vi "write_signal.vi"(6 "Experiment Settings ID":i32, 7 "Index":i32, 8 "error in":errorcluster, 9 "File Name":string="\\", 10 "Save Path":path, 11 "Signal array":T1[](array[typedef])) -> (0 "error out":errorcluster)   [LabVIEW 2012]
uses:
  Public API/Signal.ctl
  Role ID.ctl
  Hardware ID.ctl
panel:
  out "concatenated string":string
  # "Signal"
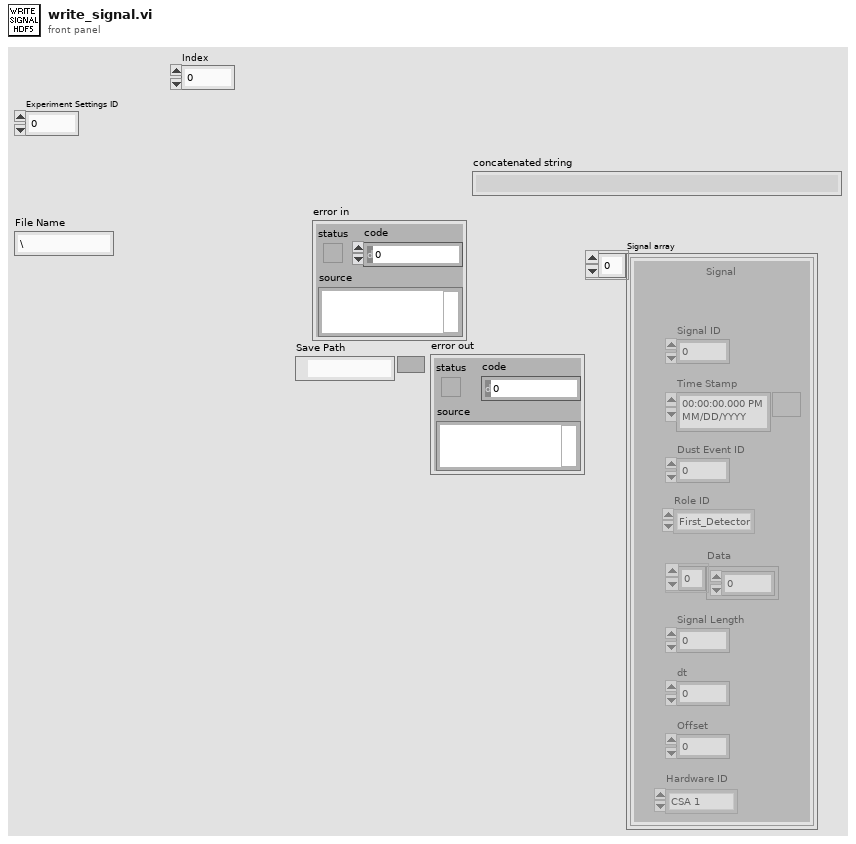
[diagram p1: front panel]
types:
  T1 = typedef "Signal.ctl" = cluster{"Signal ID":i64, "Time Stamp":timestamp, "Dust Event ID":i64, "Role ID":T2, "Data":sgl[], "Signal Length":i32, "dt":sgl, "Offset":dbl, "Hardware ID":T3}
  T2 = typedef "Role ID.ctl" = enum16{"First_Detector", "Second_Detector", "Third_Detector", "LeCroy_CH1", "LeCroy_CH2", "LeCroy_CH3", "LeCroy_CH4", "PSU"}
  T3 = typedef "Hardware ID.ctl" = enum16{"Unknown", "CSA 1", "CSA 2", "CSA 3", "CSA 4", "CSA 5", "CSA 6"}
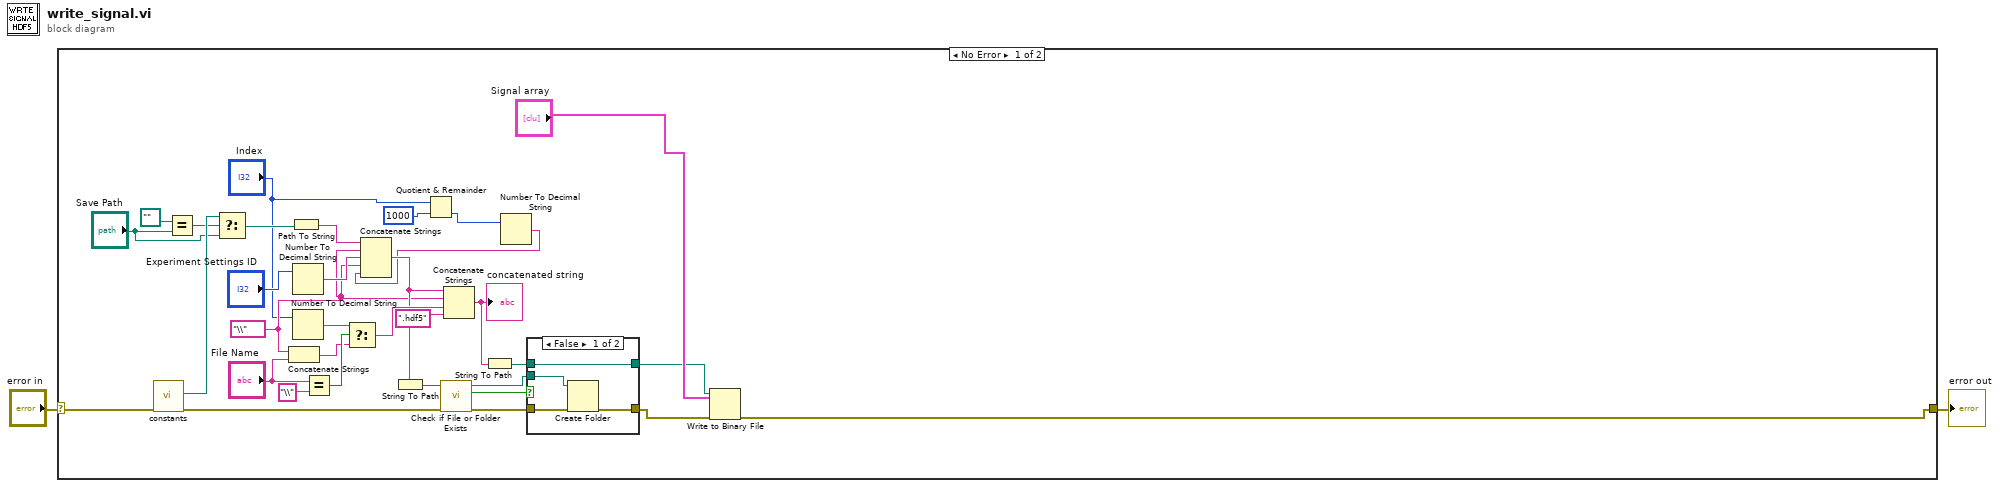
[diagram p0: block diagram]
diagram:
  n1 = case shown="No Error" "error in" {
    selector: "error in" -> [w33 w42]
    tunnel: [w3 w42] -> w1
    frame No Error {
      w11 = "\\"
      n2 = call "constants.vi"("error in (no error)"=w33) -> ("error out"=w15:errorcluster, "file path for Signal .hdf5 files"=w30:path)  [unwired: 4 in, 5 out]
      n3 = Equal?(x=path "" ("Save Path"), y="Save Path") -> (x = y?=w29:bool)
      n4 = Select(t=w30, s=w29, f="Save Path") -> (s? t:f=w32:path)
      n5 = Concatenate Strings(w11, "File Name") -> (w25:string)
      n6 = Path To String(path=w32) -> (string=w19:string)
      n7 = Number To Decimal String(number="Experiment Settings ID") -> (decimal integer string=w20:string)  [unwired: 1 in]
      n8 = Number To Decimal String(number="Index") -> (decimal integer string=w23:string)  [unwired: 1 in]
      n9 = Equal?(x="File Name", y="\\") -> (x = y?=w26:bool)
      n10 = Select(t=w23, s=w26, f=w25) -> (s? t:f=w22:string)
      n11 = Quotient & Remainder(x="Index", y=1000) -> (floor(x/y)=w8:i32)  [unwired: 1 out]
      n12 = Number To Decimal String(number=w8) -> (decimal integer string=w7:string)  [unwired: 1 in]
      n13 = Concatenate Strings(w19, w11, w20, w11, w7) -> (w14:string)
      n14 = String To Path(string=w14) -> (path=w13:path)
      n15 = call <vilib>:"Check if File or Folder Exists.vi"("error in (no error)"=w15, "path"=w13) -> ("error out"=w16:errorcluster, "file or folder exists?"=w18:bool, "dup path"=w17:path)  [unwired: 7 in]
      n16 = Concatenate Strings(w14, w11, w22, ".hdf5") -> (w35:string)
      "concatenated string" <- w35
      n17 = String To Path(string=w35) -> (path=w12:path)
      n18 = case shown="False" w18 {
        tunnel: w17 -> [w39 _]
        tunnel: w16 -> [w38 w41]
        tunnel: [w37 w41] -> w5
        tunnel: w12 -> [w36 w40]
        tunnel: [w36 w40] -> w4
        frame False {
          n19 = Create Folder(path (use dialog)=w39, error in=w38) -> (error out=w37:errorcluster)  [unwired: 1 in, 2 out]
        }
        frame True {
        }
      }
      n20 = Write to Binary File(file (use dialog)=w4, data="Signal array", error in=w5) -> (error out=w3:errorcluster)  [unwired: 3 in, 2 out]
    }
    frame Error {
    }
  }
  "error out" <- w1
